vi "Read cellStyle.vi"(8 "error in (no error)":errorcluster, 11 "CellStyle in":refnum<class "CellStyle.lvclass">) -> (0 "error out":errorcluster, 2 "cellStyle":refnum<k24>, 3 "CellStyle out":refnum<class "CellStyle.lvclass">)   [LabVIEW 2013, in "DataGrid.lvlib" / "CellStyle.lvclass"]
uses:
  CellStyle.lvclass
  System.Windows.Forms
  CellStyle.lvclass/CellStyle.ctl
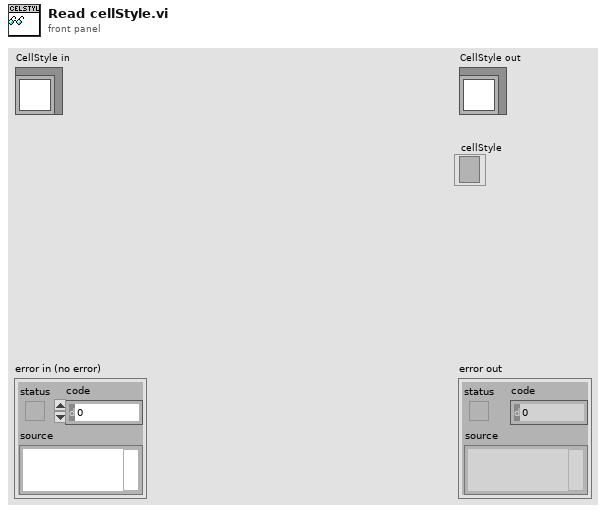
[diagram p1: front panel]
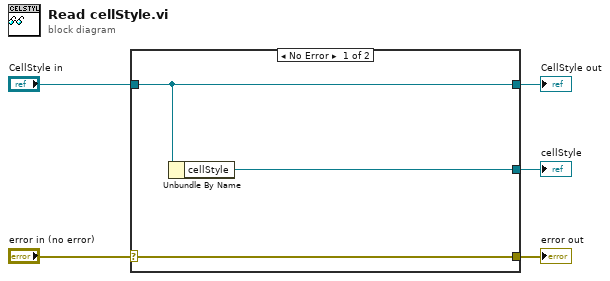
[diagram p0: block diagram]
diagram:
  n1 = case shown="No Error" "error in (no error)" {
    selector: "error in (no error)" -> [w8 w9]
    tunnel: [w8 w9] -> w4
    tunnel: [w7 w10] -> w2
    tunnel: "CellStyle in" -> [w7 w10]
    tunnel: [w6 _] -> w1
    frame No Error {
      n2 = Unbundle By Name(w7) -> ("cellStyle"=w6:refnum<k24>)
    }
    frame Error {
    }
  }
  "error out" <- w4
  "CellStyle out" <- w2
  "cellStyle" <- w1
